vi "Stop.vi"(8 "error in (no error)":errorcluster, 10 "Message in":refnum<class "StopMessage.lvclass">, 11 "Retiga in":refnum<class "Retiga.lvclass">) -> (0 "error out":errorcluster, 3 "Retiga out":refnum<class "Retiga.lvclass">)   [LabVIEW 2012, in "Retiga.lvclass"]
doc: "This member function is called when the statemachine in the run.vi receives an 'stop' command. It relays the message to all observers of the component.\n\nOverride this member function in your derived class if you need additional stop functionality (but don't forget to call the parent method)."
uses:
  Retiga.lvclass
  <vilib>/Distrio/Murmex/StopMessage/StopMessage.lvclass
  <vilib>/Distrio/Murmex/Murmex/Murmex.lvclass
panel:
  # "This method is called when the STOP\ntrigger is sent. \n\nOverride this method when your component needs to\nrespond to this trigger. \n\nCall parent for proper implementation"
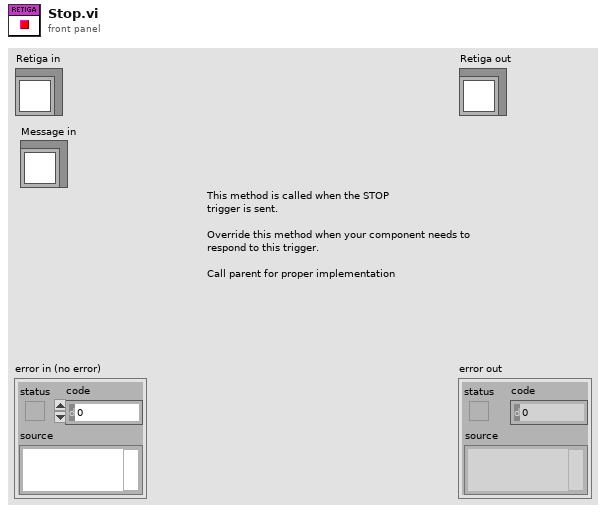
[diagram p1: front panel]
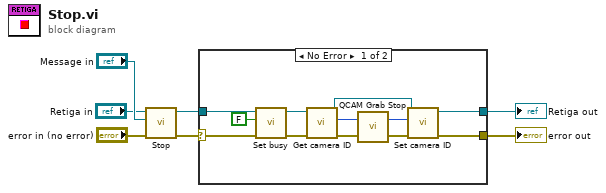
[diagram p0: block diagram]
diagram:
  n1 = call-parent "Stop.vi"("error in (no error)"="error in (no error)", "Message in"="Message in", "Murmex in"="Retiga in") -> ("error out"=w4:errorcluster, "Murmex out"=w1:refnum<class "Retiga.lvclass">)  [unwired: 7 in]
  n2 = case shown="No Error" w4 {
    selector: w4 -> [w19 w21]
    tunnel: [w15 w21] -> w3
    tunnel: [w11 w20] -> w2
    tunnel: w1 -> [w14 w20]
    frame No Error {
      n3 = call-dynamic "Set busy.vi"("error in (no error)"=w19, "busy?"=FALSE, "Retiga in"=w14) -> ("error out"=w18:errorcluster, "Retiga out"=w13:refnum<class "Retiga.lvclass">)  [unwired: 7 in]
      n4 = call-dynamic "Get camera ID.vi"("error in (no error)"=w18, "Retiga in"=w13) -> ("error out"=w17:errorcluster, "camera ID"=w10:u32, "Retiga out"=w12:refnum<class "Retiga.lvclass">)  [unwired: 7 in]
      n5 = call <userlib>:"QCAM Grab Stop.vi"("error in (no error)"=w17, "cameraId"=w10) -> ("error out"=w16:errorcluster, "cameraId Out"=w9:u32)
      n6 = call-dynamic "Set camera ID.vi"("error in (no error)"=w16, "camera ID"=w9, "Retiga in"=w12) -> ("error out"=w15:errorcluster, "Retiga out"=w11:refnum<class "Retiga.lvclass">)  [unwired: 7 in]
    }
    frame Error {
    }
  }
  "error out" <- w3
  "Retiga out" <- w2
